vi "AddDataType To Test.vi"() -> ()   [LabVIEW 2009]
uses:
  Polymorphizer+ Data Type.ctl
  <userlib>/_OpenG.lib/array/array.llb/Remove Duplicates from 1D Array (I16)__ogtk.vi
panel:
  out "Test Cases updated":i32
  in  "Data Type(s) to add":T1[](array[typedef])=[enum."LabVIEW Object"]
  in  "Cluster Element Name":string
  in  "Control":string
  in  "VI name":string
  # "Instructions:\n1:Open a VI to add a datatype to\n2:Set the VI Name, Control name and Cluster element name\n3: Select the Datatype to Add\n4: Run this VI\n5: Adjust the BD of the Test VI with a test for the new datatype\n6: Save the Test VI"
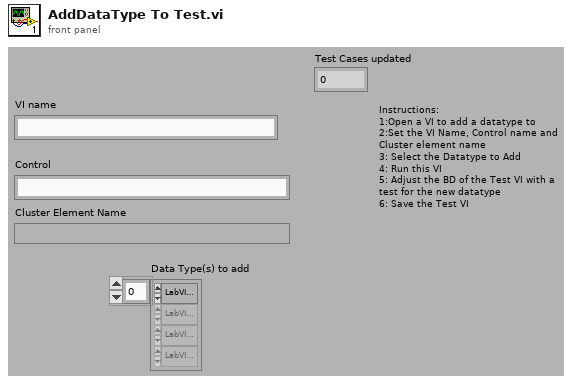
[diagram p1: front panel]
types:
  T1 = typedef "Polymorphizer+ Data Type.ctl" = enum16{"EXT", "DBL", "SGL", "I32", "I16", "I8", "U32", "U16", "U8", "CXT", "CDB", "CSG", "Boolean", "String", "Path", "Variant", "CTL-REF", "GEN-REF", "GObj-REF", "VI-REF", "ENUM", "ERR", "FILE-REF", "MENU-REF", "MENU-RING", "PICT-RING", "TXT&PICT-RING", "TXT-RING", "I64", "U64", "LabVIEW Object"}
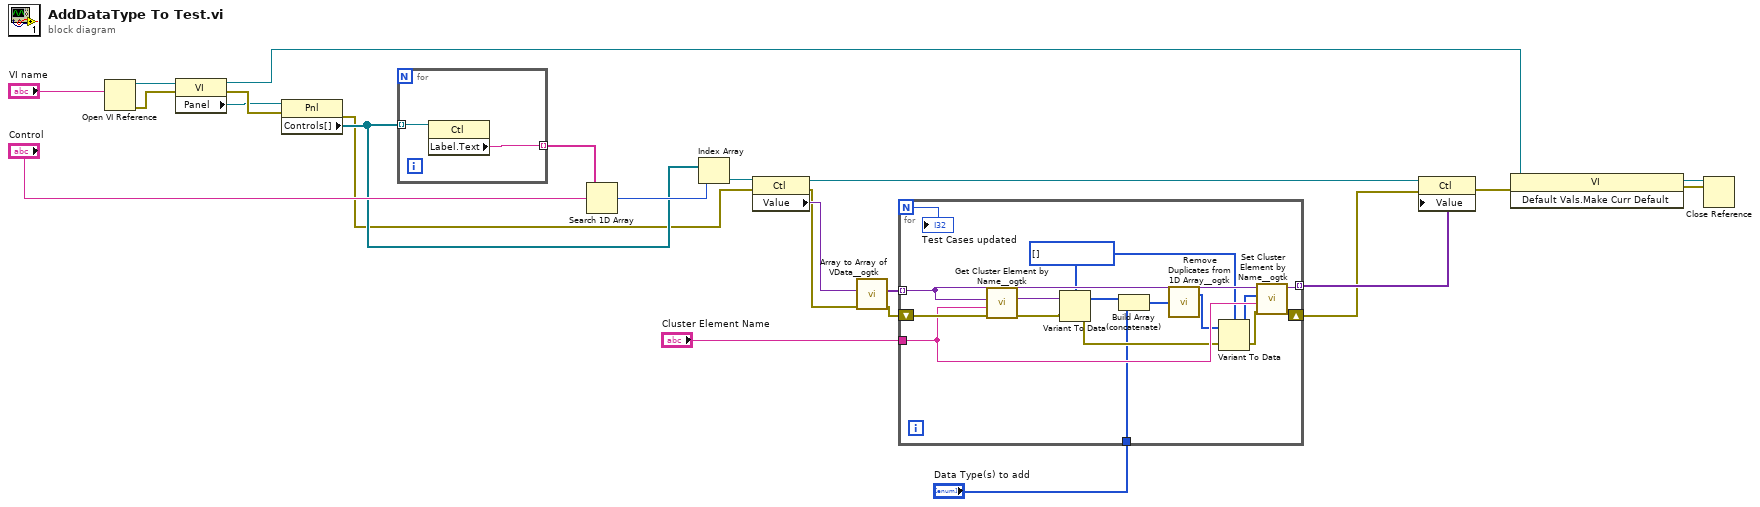
[diagram p0: block diagram]
diagram:
  n1 = Open VI Reference(vi path="VI name") -> (vi reference=w23:refnum<vi>, error out=w22:errorcluster)  [unwired: 5 in]
  n2 = property class="VI"(reference=w23, error in=w22) -> (reference out=w2:refnum<vi>, error out=w21:errorcluster, "Panel"=w4:refnum<vi>)
  n3 = property class="Pnl"(reference=w4, error in=w21) -> (error out=w15:errorcluster, "Controls[]"=w17:refnum<vi>[])  [unwired: 1 out]
  n4 = for {
    tunnel: w17 -> [w26] mode=indexing
    tunnel: [w25] -> w20 mode=indexing
    n5 = property class="Ctl"(reference=w26) -> ("Label.Text"=w25:string)  [unwired: 1 in, 2 out]
  }
  n6 = Search 1D Array(1D array=w20, element="Control") -> (index of element=w18:i32)  [unwired: 1 in]
  n7 = Index Array(array=w17, index=w18) -> (element=w16:refnum<vi>)
  n8 = property class="Ctl"(reference=w16, error in=w15) -> (reference out=w8:refnum<vi>, error out=w12:errorcluster, "Value"=w14:variant)
  n9 = call <userlib>:"Array to Array of VData__ogtk.vi"("error in (no error)"=w12, "MultiD Array"=w14) -> ("error out"=w11:errorcluster, "1D Array of Variants"=w13:variant[])  [unwired: 8 in]
  n10 = for {
    N -> [w27]
    tunnel: w13 -> [w38] mode=indexing
    shift-right: [w36] -> w7
    shift-left: w11 -> [w42]
    tunnel: "Cluster Element Name" -> [w37]
    tunnel: [w35] -> w9 mode=indexing
    tunnel: "Data Type(s) to add" -> [w28]
    w31 = T1[] [] items=["EXT", "DBL", "SGL", "I32", "I16", "I8", "U32", "U16", "U8", "CXT", "CDB", "CSG", "Boolean", "String", "Path", "Variant", "CTL-REF", "GEN-REF", "GObj-REF", "VI-REF", "ENUM", "ERR", "FILE-REF", "MENU-REF", "MENU-RING", "PICT-RING", "TXT&PICT-RING", "TXT-RING", "I64", "U64", "LabVIEW Object"]
    n11 = call <userlib>:"Get Cluster Element by Name__ogtk.vi"("error in (no error)"=w42, "Element Name"=w37, "Cluster"=w38) -> ("error out"=w40:errorcluster, "VElement"=w41:variant)  [unwired: 6 in, 1 out]
    n12 = Variant To Data(error in=w40, Variant=w41, type=w31) -> (error out=w30:errorcluster, data=w39:T1[])
    n13 = Build Array (concatenate)(w39, w28) -> (w34:T1[])
    n14 = call-poly <userlib>:"Remove Duplicates from 1D Array__ogtk.vi"("Input Array"=w34) -> ("Output Array"=w33:i16[])  [unwired: 1 out]
    n15 = Variant To Data(error in=w30, Variant=w33, type=w31) -> (error out=w29:errorcluster, data=w32:T1[])
    n16 = call <userlib>:"Set Cluster Element by Name__ogtk.vi"("error in (no error)"=w29, "Element Name (\"\": New Element Data Name)"=w37, "New Element Value"=w32, "Cluster"=w38) -> ("error out"=w36:errorcluster, "VCluster out"=w35:variant)  [unwired: 5 in, 1 out]
    "Test Cases updated" <- w27
  }
  n17 = property class="Ctl"(reference=w8, error in=w7, "Value"=w9) -> (error out=w6:errorcluster)  [unwired: 1 out]
  n18 = invoke class="VI" method="Default Vals.Make Curr Default"(reference=w2, error in=w6) -> (reference out=w5:refnum<vi>, error out=w3:errorcluster)  [unwired: 1 in, 1 out]
  n19 = Close Reference(reference=w5, error in (no error)=w3) -> ()  [unwired: 1 out]
